vi "声发射_RMS.vi"(11 "输入信号":dbl[](array[numeric])=[0.0, 1.0, 0.0, 4.0, 0.0, 4.0, 0.0, 1.0, 0.0, 3.0, 0.0, 4.0, 0.0, 1.0, 0.0, 2.0, 3.0] caption="X") -> (3 "RMS value":dbl caption="RMS" format="%0.5f")   [LabVIEW 2014]
uses:
  <vilib>/measure/madcrms.llb/Basic Averaged DC-RMS for 1 Chan.vi
  <vilib>/measure/NI_MAPro.lvlib
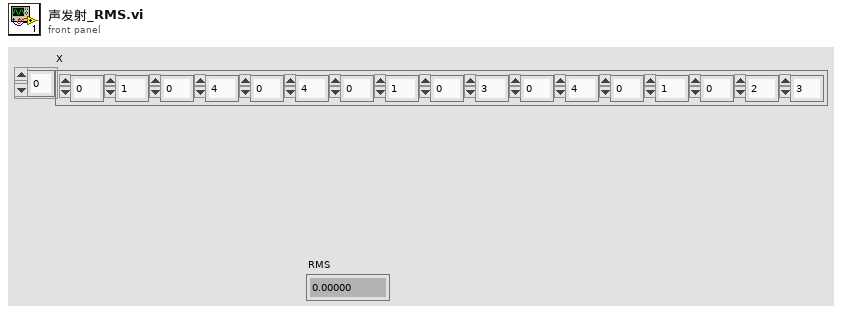
[diagram p1: front panel]
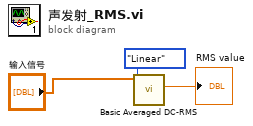
[diagram p0: block diagram]
diagram:
  n1 = call-poly <vilib>:"Basic Averaged DC-RMS.vi"("averaging type"=enum16{"Linear", "Exponential"}."Linear", "signal in"="输入信号") -> ("RMS value"=→"RMS value":dbl)  [unwired: 6 in, 3 out]
